vi "Main2.vi"() -> ()   [LabVIEW 2017]
doc: "The myRIO Project template acquires acceleration data from the onboard accelerometer and displays the changes of acceleration values in a waveform chart."
uses:
  Control 2.ctl
  <vilib>/myRIO/Instrument Drivers/Onboard IO/DIO/typedefs/DIO Reference.ctl
  <vilib>/myRIO/Common/Instrument Driver Framework/Utilities/typedefs/myRIO Generic Hardware Reference.ctl
  <vilib>/myRIO/Common/Instrument Driver Framework/Utilities/typedefs/Hardware Version Enum.ctl
  <vilib>/myRIO/Common/Instrument Driver Framework/Utilities/typedefs/myRIO v1.0 Reference.ctl
  <vilib>/myRIO/Common/Instrument Driver Framework/Utilities/typedefs/Generic FPGA Reference.ctl
  <vilib>/myRIO/Common/Instrument Driver Framework/myRIO v1.0/DIO/typedefs/DIO Channels List.ctl
  <vilib>/myRIO/Common/Instrument Driver Framework/myRIO v1.0/DIO/typedefs/DIO Channels Enum.ctl
  <vilib>/userdefined/High Color/nirio_resource_hc.ctl
  <vilib>/myRIO/Common/Instrument Driver Framework/Utilities/vis/Is FPGA Ref Available.vi
  <vilib>/myRIO/Common/Instrument Driver Framework/myRIO v1.0/DIO/vis/myRIO v1.1 Open DIO.vi
  <vilib>/myRIO/Instrument Drivers/Onboard IO/DIO/vis/Write.vi
  <vilib>/myRIO/Common/Instrument Driver Framework/Utilities/vis/Validate Channels.vi
  <vilib>/myRIO/Common/Instrument Driver Framework/myRIO v1.0/DIO/vis/myRIO v1.0 Reserve DIO.vi
  <vilib>/myRIO/Common/Instrument Driver Framework/myRIO v1.0/UART/vis/myRIO v1.0 Close UART.vi
  <vilib>/myRIO/Common/Instrument Driver Framework/myRIO v1.0/Resource Manager/vis/myRIO v1.0 Reserve Channel List.vi
  <vilib>/myRIO/Common/Instrument Driver Framework/myRIO v1.0/DIO/vis/myRIO v1.0 Build MUX Configuration DIO.vi
  <vilib>/myRIO/Common/Instrument Driver Framework/myRIO v1.0/Resource Manager/vis/myRIO v1.0 Reserve Channel.vi
  <vilib>/myRIO/Common/Instrument Driver Framework/myRIO v1.0/Resource Manager/vis/myRIO v1.0 Unreserve Channel.vi
  <vilib>/myRIO/Common/Instrument Driver Framework/myRIO v1.0/Resource Manager/vis/myRIO v1.0 Create Configuration List.vi
  <vilib>/myRIO/Common/Instrument Driver Framework/myRIO v1.0/Resource Manager/vis/myRIO v1.0 Build Mutex Name.vi
  Globales.vi
  <vilib>/Utility/VariantDataType/GetNumericInfo.vi
  <vilib>/Utility/error.llb/Error Cluster From Error Code.vi
  <vilib>/myRIO/Common/Instrument Driver Framework/myRIO v1.0/myRIO v1.1 Open.vi
  <vilib>/myRIO/Common/Instrument Driver Framework/Utilities/vis/IO Manager.vi
  <vilib>/myRIO/Common/Instrument Driver Framework/Utilities/vis/Configuration Manager.vi
  <vilib>/myRIO/Common/Instrument Driver Framework/myRIO v1.0/Resource Manager/vis/myRIO v1.0 Configure IO.vi
  <vilib>/myRIO/Common/Instrument Driver Framework/myRIO v1.0/myRIO v1.0 Close.vi
  <vilib>/myRIO/Common/Instrument Driver Framework/myRIO v1.0/DIO/vis/myRIO v1.0 Write DIO.vi
  <vilib>/myRIO/Common/Instrument Driver Framework/Utilities/vis/FPGA Ref Manager.vi
  <vilib>/myRIO/Common/Instrument Driver Framework/myRIO v1.0/myRIO v1.0 Reset FPGA.vi
  <vilib>/myRIO/Common/Instrument Driver Framework/myRIO v1.0/IRQ/vis/myRIO v1.0 IRQ Info FGV.vi
  <vilib>/myRIO/Common/Instrument Driver Framework/myRIO v1.0/IRQ/vis/myRIO v1.0 Timer IRQ Info FGV.vi
  <vilib>/myRIO/Common/Instrument Driver Framework/myRIO v1.0/IRQ/vis/myRIO v1.0 ISR Agent.vi
  <vilib>/myRIO/Express VI/Onboard IO/DO/DO Express VI.xnode
  <vilib>/myRIO/Instrument Drivers/Onboard IO/DIO/vis/myRIO DIO Open.xnode
  <vilib>/myRIO/Instrument Drivers/Utilities/Utilities.lvlib
  <vilib>/myRIO/Instrument Drivers/Onboard IO/DIO/DIO.lvlib
panel:
  in  "RangoY":dbl
  in  "RangoX":dbl
  in  "Avance_Calibrar":dbl
  in  "RelY":dbl
  in  "RelX":dbl
  in  "Avance Medición":dbl
  in  "Alto":dbl
  in  "Ancho":dbl
  in  "Medir":bool
  out "RelY":dbl
  out "RelX":dbl
  out "Posición en Y":dbl
  in  "Posición":T1
  in  "Negativo_Y":bool
  in  "Positivo_Y":bool
  in  "Calibrar":bool
  in  "Home":bool
  in  "Ir_posicion":bool
  out "Posición en X":dbl
  in  "Positivo_X":bool
  in  "Negativo_X":bool
  in  "Avance":dbl
  out "error out":errorcluster
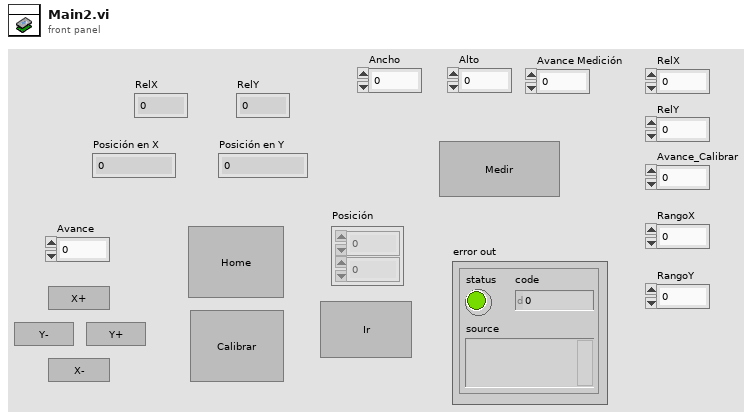
[diagram p1: front panel]
types:
  T1 = typedef "Control 2.ctl" = dbl[]
  T2 = typedef "DIO.lvlib/DIO Reference.ctl" = cluster{"myRIO Reference":T3, "DIO Channels List":T7}
  T3 = typedef "myRIO Generic Hardware Reference.ctl" = cluster{"myRIO Model":T4, "myRIO Hardware Reference":T5}
  T4 = typedef "Hardware Version Enum.ctl" = enum16{"Unknown", "myRIO-1900", "myRIO-1950", "roboRIO", "NI ELVIS RIO CM"}
  T5 = typedef "myRIO v1.0 Reference.ctl" = cluster{"Generic FPGA Reference":T6, "Allow multiple opens":bool}
  T6 = typedef "Generic FPGA Reference.ctl" = refnum<k20>
  T7 = typedef "DIO Channels List.ctl" = T8[]
  T8 = typedef "DIO Channels Enum.ctl" = enum16{"Not Connected", "C/DIO0", "C/DIO1", "C/DIO2", "C/DIO3", "C/DIO4", "C/DIO5", "C/DIO6", "C/DIO7", "A/DIO0", "A/DIO1", "A/DIO2", "A/DIO3", "A/DIO4", "A/DIO5", "A/DIO6", "A/DIO7", "A/DIO8", "A/DIO9", "A/DIO10", "A/DIO11", "A/DIO12", "A/DIO13", "A/DIO14", "A/DIO15", "B/DIO0", "B/DIO1", "B/DIO2", "B/DIO3", "B/DIO4", "B/DIO5", "B/DIO6", "B/DIO7", "B/DIO8", "B/DIO9", "B/DIO10", "B/DIO11", "B/DIO12", "B/DIO13", "B/DIO14", "B/DIO15", "LED0", "LED1", "LED2", "LED3", "Button0", "DIO/DIO0", "DIO/DIO1", "DIO/DIO2", "DIO/DIO3", "DIO/DIO4", "DIO/DIO5", "DIO/DIO6", "DIO/DIO7", "DIO/DIO8", "DIO/DIO9", "SPI/CS0", "SPI/CS1", "SPI/CS2", "SPI/CS3", "LED RADIO (Green)", "LED RADIO (Red)", "LED COMM (Green)", "LED COMM (Red)", "LED MODE (Green)", "LED MODE (Red)"}
  T9 = typedef "nirio_resource_hc.ctl" = tag
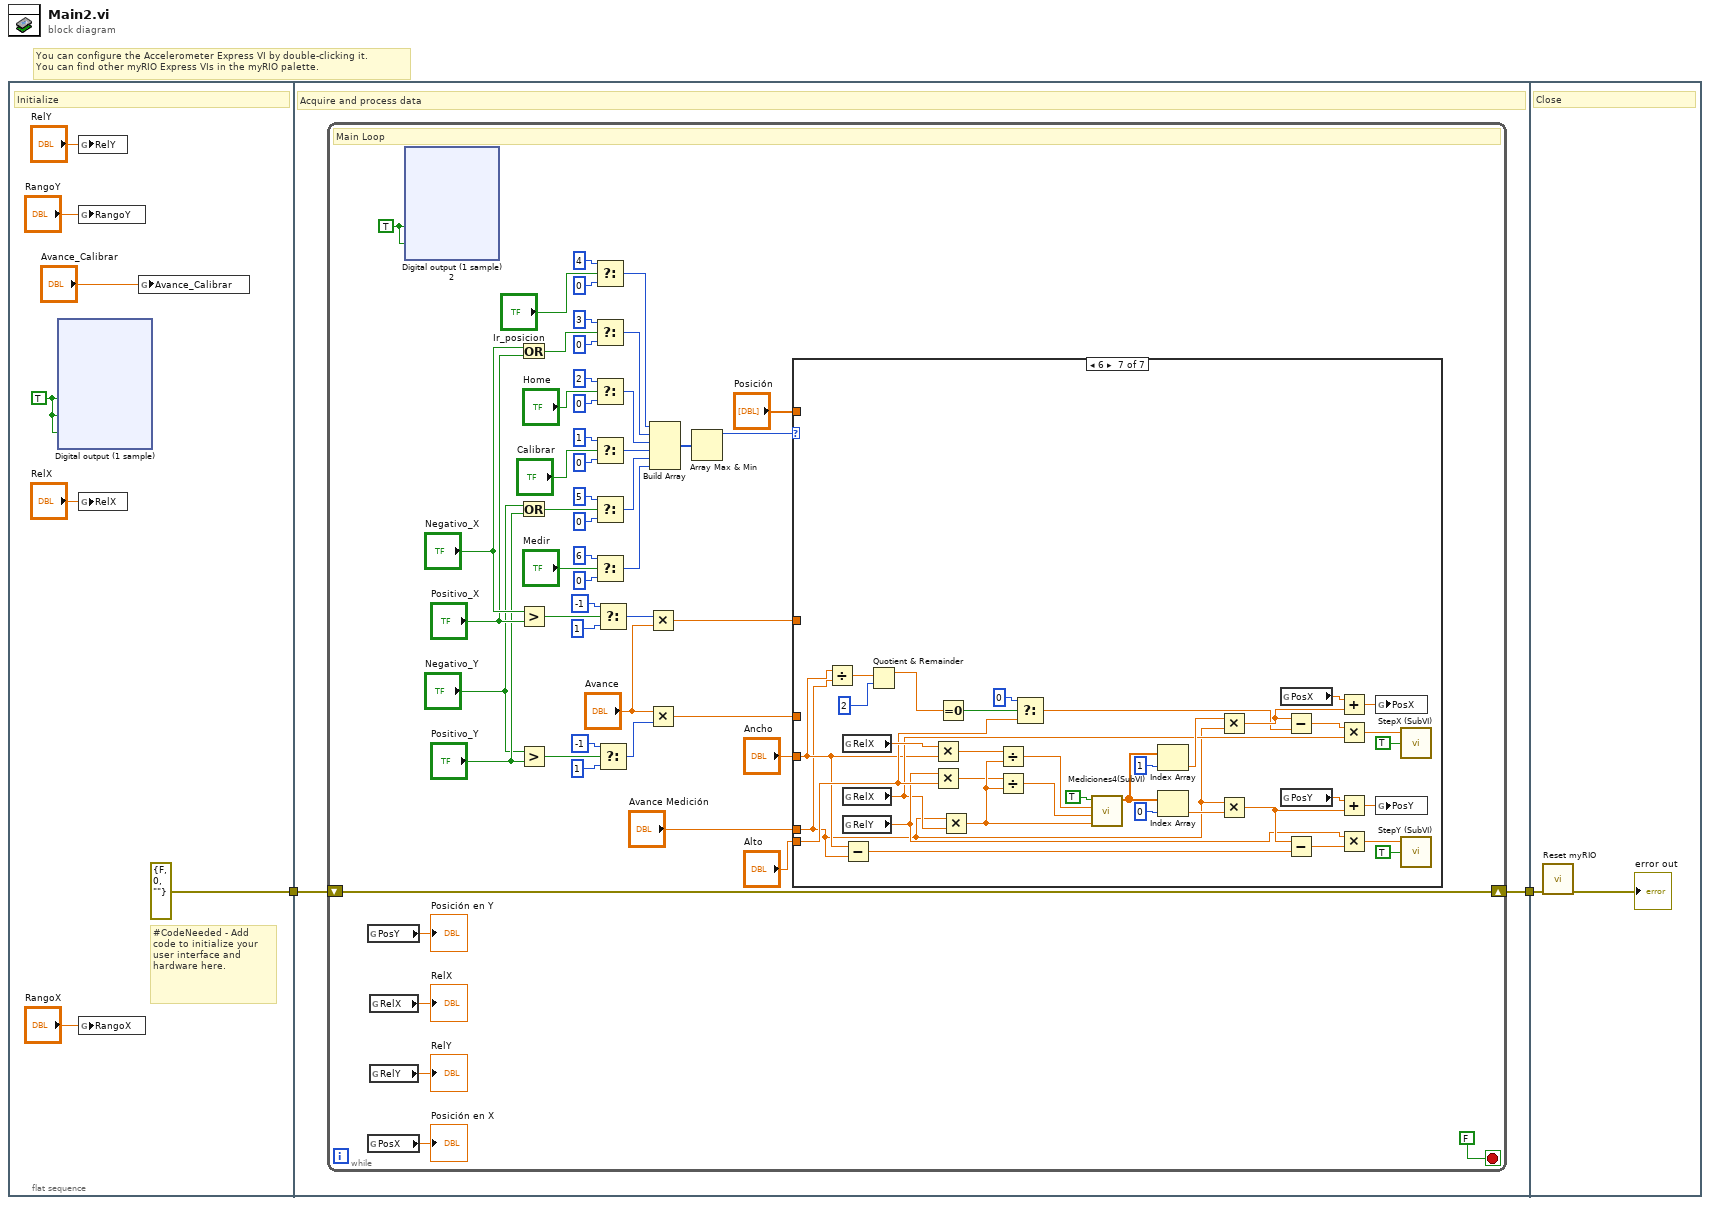
[diagram p0: block diagram]
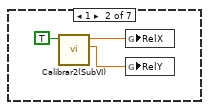
[diagram p3: hidden frame]
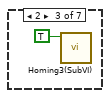
[diagram p4: hidden frame]
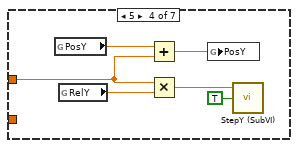
[diagram p5: hidden frame]
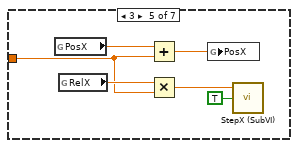
[diagram p6: hidden frame]
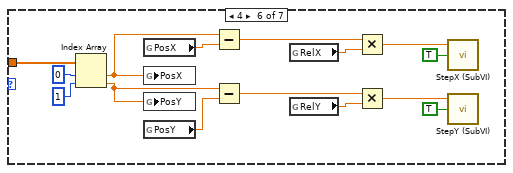
[diagram p7: hidden frame]
diagram:
  # "You can configure the Accelerometer Express VI by double-clicking it.\nYou can find other myRIO Express VIs in the myRIO palette."
  n1 = flat-sequence {
    tunnel: [errorcluster {"status"=FALSE, "code"=0, "source"=""} ("error in (no error)")] -> w2
    tunnel: w2 -> [w48]
    tunnel: [w47] -> w1
    tunnel: w1 -> [w205]
    frame #0 {
      w8 = TRUE
      # "#CodeNeeded - Add code to initialize your user interface and hardware here."
      # "Initialize"
      n2 = xnode "Digital output (1 sample)"("Direccion (A/DIO0 (Pin 11))"=w8, "Step (A/DIO1 (Pin 13))"=w8, "ON/OFF (A/DIO4 (Pin 19))"=w8) -> ()  [unwired: 1 in, 1 out]
      n3 = global write "Globales.vi" "RelY"("RelY") -> ()
      n4 = global write "Globales.vi" "RangoY"("RangoY") -> ()
      n5 = global write "Globales.vi" "RelX"("RelX") -> ()
      n6 = global write "Globales.vi" "RangoX"("RangoX") -> ()
      n7 = global write "Globales.vi" "Avance_Calibrar"("Avance_Calibrar") -> ()
    }
    frame #1 {
      # "Acquire and process data"
      n8 = while {
        shift-right: [w77] -> w47
        shift-left: w48 -> [w77]
        stop <- FALSE stop-if-true
        w59 = TRUE
        # "Main Loop"
        n9 = global read "Globales.vi" "PosY"() -> (→"Posición en Y":dbl)
        n10 = global read "Globales.vi" "PosX"() -> (→"Posición en X":dbl)
        n11 = global read "Globales.vi" "RelX"() -> (→"RelX":dbl)
        n12 = global read "Globales.vi" "RelY"() -> (→"RelY":dbl)
        n13 = xnode "Digital output (1 sample) 2"("ON/OFF X (A/DIO4 (Pin 19))"=w59, "ON/OFF Y (A/DIO7 (Pin 25))"=w59) -> ()  [unwired: 1 in, 1 out]
        n14 = Or(x="Negativo_X", y="Positivo_X") -> (x .or. y?=w90:bool)
        n15 = Or(x="Negativo_Y", y="Positivo_Y") -> (x .or. y?=w70:bool)
        n16 = Greater?(x="Negativo_X", y="Positivo_X") -> (0:w80:bool)
        n17 = Greater?(x="Negativo_Y", y="Positivo_Y") -> (0:w66:bool)
        n18 = Select(t=4, s="Ir_posicion", f=0) -> (s? t:f=w88:i32)
        n19 = Select(t=3, s=w90, f=0) -> (s? t:f=w87:i32)
        n20 = Select(t=2, s="Home", f=0) -> (s? t:f=w86:i32)
        n21 = Select(t=1, s="Calibrar", f=0) -> (s? t:f=w85:i32)
        n22 = Select(t=5, s=w70, f=0) -> (s? t:f=w69:i32)
        n23 = Select(t=6, s="Medir", f=0) -> (s? t:f=w55:i32)
        n24 = Select(t=-1, s=w80, f=1) -> (s? t:f=w61:i32)
        n25 = Select(t=-1, s=w66, f=1) -> (s? t:f=w63:i32)
        n26 = Multiply(x=w61, y="Avance") -> (x*y=w75:dbl)
        n27 = Multiply(x="Avance", y=w63) -> (x*y=w62:dbl)
        n28 = Build Array(w88, w87, w86, w85, w69, w55) -> (w84:i32[])
        n29 = Array Max & Min(array=w84) -> (max value=w83:i32)  [unwired: 3 out]
        n30 = case shown="6" w83 {
          tunnel: w75 -> [_ _ _ _ w149 _ _]
          tunnel: "Posición" -> [_ _ _ _ _ w167 _]
          tunnel: w62 -> [_ _ _ w141 _ _ _]
          tunnel: "Ancho" -> [_ _ _ _ _ _ w171]
          tunnel: "Alto" -> [_ _ _ _ _ _ w178]
          tunnel: "Avance Medición" -> [_ _ _ _ _ _ w170]
          frame 0, Default {
          }
          frame 1 {
            n31 = call "Calibrar2(SubVI).vi"("Calibrar"=TRUE) -> ("Relación2"=w138:dbl, "Relación"=w139:dbl)  [unwired: 9 in]
            n32 = global write "Globales.vi" "RelX"(w139) -> ()
            n33 = global write "Globales.vi" "RelY"(w138) -> ()
          }
          frame 2 {
            n34 = call "Homing3(SubVI).vi"("Home"=TRUE) -> ()  [unwired: 10 in, 1 out]
          }
          frame 5 {
            n35 = global read "Globales.vi" "PosY"() -> (w146:dbl)
            n36 = global read "Globales.vi" "RelY"() -> (w142:dbl)
            n37 = Add(x=w146, y=w141) -> (x+y=w145:dbl)
            n38 = Multiply(x=w141, y=w142) -> (x*y=w144:dbl)
            n39 = global write "Globales.vi" "PosY"(w145) -> ()
            n40 = call "StepY (SubVI).vi"("Mover"=TRUE, "Step"=w144) -> ()  [unwired: 3 in]
          }
          frame 3 {
            n41 = global read "Globales.vi" "PosX"() -> (w150:dbl)
            n42 = global read "Globales.vi" "RelX"() -> (w152:dbl)
            n43 = Add(x=w150, y=w149) -> (x+y=w151:dbl)
            n44 = Multiply(x=w152, y=w149) -> (x*y=w148:dbl)
            n45 = global write "Globales.vi" "PosX"(w151) -> ()
            n46 = call "StepX (SubVI).vi"("Mover"=TRUE, "Step"=w148) -> ()  [unwired: 3 in]
          }
          frame 4 {
            n47 = Index Array(array=w167, index #1=0, index #2=1) -> (element #1=w153:dbl, element #2=w154:dbl)
            n48 = global read "Globales.vi" "PosX"() -> (w164:dbl)
            n49 = global write "Globales.vi" "PosX"(w153) -> ()
            n50 = global write "Globales.vi" "PosY"(w154) -> ()
            n51 = global read "Globales.vi" "PosY"() -> (w159:dbl)
            n52 = Subtract(x=w153, y=w164) -> (x-y=w163:dbl)
            n53 = Subtract(x=w154, y=w159) -> (x-y=w158:dbl)
            n54 = global read "Globales.vi" "RelX"() -> (w162:dbl)
            n55 = global read "Globales.vi" "RelY"() -> (w157:dbl)
            n56 = Multiply(x=w163, y=w162) -> (x*y=w161:dbl)
            n57 = Multiply(x=w158, y=w157) -> (x*y=w156:dbl)
            n58 = call "StepX (SubVI).vi"("Mover"=TRUE, "Step"=w161) -> ()  [unwired: 3 in]
            n59 = call "StepY (SubVI).vi"("Mover"=TRUE, "Step"=w156) -> ()  [unwired: 3 in]
          }
          frame 6 {
            n60 = Divide(x=w171, y=w170) -> (x/y=w169:dbl)
            n61 = global read "Globales.vi" "RelX"() -> (w202:dbl)
            n62 = global read "Globales.vi" "RelX"() -> (w173:dbl)
            n63 = global read "Globales.vi" "RelY"() -> (w174:dbl)
            n64 = Subtract(x=w171, y=w170) -> (x-y=w182:dbl)
            n65 = Quotient & Remainder(x=w169, y=2) -> (x-y*floor(x/y)=w181:dbl)  [unwired: 1 out]
            n66 = Multiply(x=w202, y=w171) -> (x*y=w194:dbl)
            n67 = Multiply(x=w174, y=w178) -> (x*y=w188:dbl)
            n68 = Equal To 0?(x=w181) -> (x = 0?=w180:bool)
            n69 = Multiply(x=w170, y=w173) -> (x*y=w193:dbl)
            n70 = Divide(x=w194, y=w193) -> (x/y=w196:dbl)
            n71 = Divide(x=w188, y=w193) -> (x/y=w195:dbl)
            n72 = Select(t=0, s=w180, f=w178) -> (s? t:f=w176:dbl)
            n73 = call "Mediciones4(SubVI).vi"("Pasos"=w193, "Ancho"=w195, "Alto"=w196, "OK Button"=TRUE) -> ("Array"=w200:dbl[])  [unwired: 7 in]
            n74 = Index Array(array=w200, index=1) -> (element=w189:dbl)
            n75 = Index Array(array=w200, index=0) -> (element=w187:dbl)
            n76 = Multiply(x=w189, y=w170) -> (x*y=w177:dbl)
            n77 = Multiply(x=w170, y=w187) -> (x*y=w183:dbl)
            n78 = global read "Globales.vi" "PosX"() -> (w191:dbl)
            n79 = global read "Globales.vi" "PosY"() -> (w192:dbl)
            n80 = Subtract(x=w177, y=w176) -> (x-y=w175:dbl)
            n81 = Subtract(x=w183, y=w182) -> (x-y=w184:dbl)
            n82 = Add(x=w191, y=w177) -> (x+y=w190:dbl)
            n83 = Multiply(x=w175, y=w173) -> (x*y=w172:dbl)
            n84 = Add(x=w192, y=w183) -> (x+y=w186:dbl)
            n85 = Multiply(x=w174, y=w184) -> (x*y=w185:dbl)
            n86 = global write "Globales.vi" "PosX"(w190) -> ()
            n87 = global write "Globales.vi" "PosY"(w186) -> ()
            n88 = call "StepX (SubVI).vi"("Mover"=TRUE, "Step"=w172) -> ()  [unwired: 3 in]
            n89 = call "StepY (SubVI).vi"("Mover"=TRUE, "Step"=w185) -> ()  [unwired: 3 in]
          }
        }
      }
    }
    frame #2 {
      # "Close"
      n90 = call <vilib>:"Reset myRIO.vi"("error in (no error)"=w205) -> ("error out"=→"error out":errorcluster)  [unwired: 10 in]
    }
  }
